vi "Write PMUComms.vi"(8 "error in (no error)":errorcluster, 10 "PMU Comms":T1={"PMU IP Address"="192.92.92.92", "CMD Comms Type"=enum."TCP", "Data Comms Type"=enum."TCP", "CMD Port"=4712, "Data Port"=4712, "PMU ID"=1}, 11 "C37.118 PMU in":refnum<class "C37.118 PMU.lvclass">) -> (0 "error out":errorcluster, 3 "C37.118 PMU out":refnum<class "C37.118 PMU.lvclass">)   [LabVIEW 2014, in "SensorPlugins.lvlib" / "C37.118 PMU.lvclass"]
uses:
  C37.118 PMU.lvclass
  Typedef/PMUComms.ctl
  Typedef/eCommsType.ctl
  C37.118 PMU.lvclass/C37.118 PMU.ctl
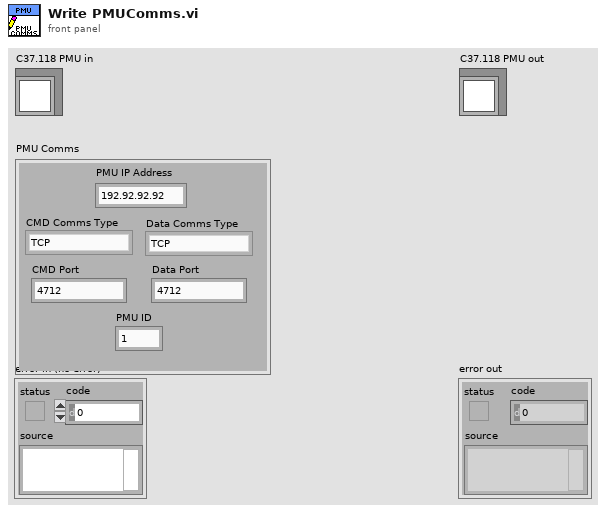
[diagram p1: front panel]
types:
  T1 = typedef "SensorPlugins.lvlib/C37.118 PMU.lvclass/PMUComms.ctl" = cluster{"PMU IP Address":string, "CMD Comms Type":T2, "Data Comms Type":T2, "CMD Port":u16, "Data Port":u16, "PMU ID":u16}
  T2 = typedef "SensorPlugins.lvlib/C37.118 PMU.lvclass/eCommsType.ctl" = enum16{"TCP", "UDP", "USB", "GPIB"}
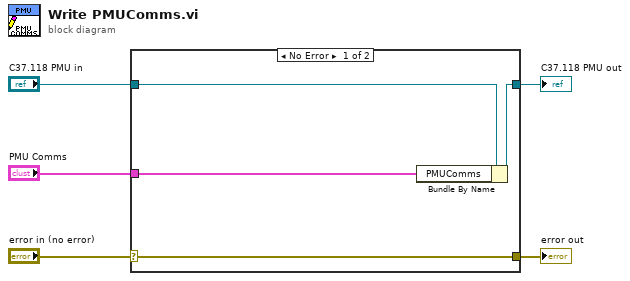
[diagram p0: block diagram]
diagram:
  n1 = case shown="No Error" "error in (no error)" {
    selector: "error in (no error)" -> [w9 w10]
    tunnel: [w9 w10] -> w4
    tunnel: [w7 w11] -> w2
    tunnel: "C37.118 PMU in" -> [w8 w11]
    tunnel: "PMU Comms" -> [w6 _]
    frame No Error {
      n2 = Bundle By Name(cluster=w8, "PMUComms"=w6) -> (w7:refnum<class "C37.118 PMU.lvclass">)
    }
    frame Error {
    }
  }
  "error out" <- w4
  "C37.118 PMU out" <- w2
